vi "Initialise_ColDet.vi"(11 "Init Panel":T1={"Width"=800, "Lock to 60Hz?"=FALSE, "Height"=600, "Camera Type"=enum."Standard Camera", "Graphics Driver Type"=enum."Software Driver"}) -> (0 "error out":errorcluster)   [LabVIEW 2011]
doc: "This VI will setup initialise the graphics requirements for the collision detection. This should be called regardless of whether graphics are required to be displayed or not, since the vertex buffers associated with the graphics are used in the collision detection algorithms."
uses:
  Enflo_Collision_Detection.dll
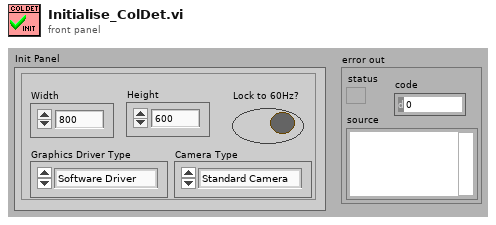
[diagram p1: front panel]
types:
  T1 = cluster{"Width":i32, "Lock to 60Hz?":bool, "Height":i32, "Camera Type":enum32{"Fixed Camera", "Standard Camera", "Flying Camera"}, "Graphics Driver Type":enum32{"No Driver (NULL)", "Software Driver", "Burnings Video", "DirectX 8", "DirectX 9", "OpenGL", "Count"}}
  T2 = enum32{"Fixed Camera", "Standard Camera", "Flying Camera"}
  T3 = enum32{"No Driver (NULL)", "Software Driver", "Burnings Video", "DirectX 8", "DirectX 9", "OpenGL", "Count"}
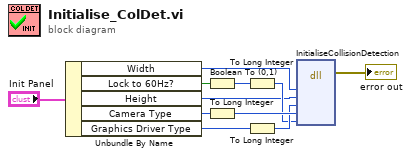
[diagram p0: block diagram]
diagram:
  n1 = Unbundle By Name("Init Panel") -> ("Width"=w5:i32, "Lock to 60Hz?"=w3:bool, "Height"=w4:i32, "Camera Type"=w1:T2, "Graphics Driver Type"=w2:T3)
  n2 = Boolean To (0,1)(Boolean=w3) -> (0, 1=w8:i16)
  n3 = To Long Integer(number=w1) -> (32bit integer=w10:i32)
  n4 = To Long Integer(number=w8) -> (32bit integer=w7:i32)
  n5 = To Long Integer(number=w2) -> (32bit integer=w9:i32)
  n6 = dll-call lib="C:/Enflo_Software_SVN/EnFloSW/Anemometry/Anemometry Sub Vis/Collision_Detection/Enflo_Collision_Detection.dll" fn="InitialiseCollisionDetection"("Width"=w5, "Height"=w4, "Graphics Driver"=w9, "Camera Type"=w10, "Vsync"=w7) -> (error out=→"error out":errorcluster)  [unwired: 9 in, 1 out]
